vi "ConvertDataSetToWfm.vi"(10 "DataSet":T1) -> (2 "waveform":waveform(sgl))   [LabVIEW 2016]
doc: "Converts a NI InsightCM data set to a waveform data type."
uses:
  <vilib>/addons/InsightCM/Utilities/PropertyHelpers/PropertyHelpers.lvlib
  <vilib>/addons/InsightCM/MessageBus/Base/controls/KeyValuePair.ctl
  <vilib>/addons/InsightCM/MessageBus/Base/controls/DataSetByteData.ctl
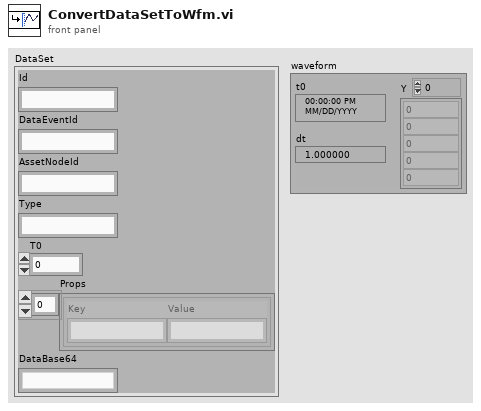
[diagram p1: front panel]
types:
  T1 = typedef "DataSetByteData.ctl" = cluster{"Id":string, "DataEventId":string, "AssetNodeId":string, "Type":string, "T0":i64, "Props":T2[], "DataBase64":string}
  T2 = typedef "KeyValuePair.ctl" = cluster{"Key":string, "Value":string}
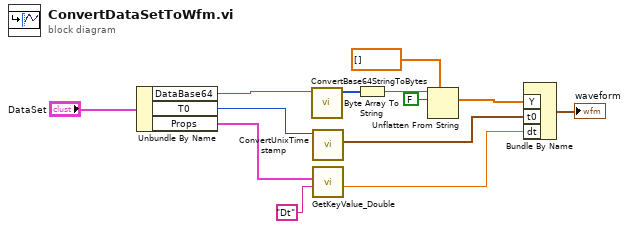
[diagram p0: block diagram]
diagram:
  n1 = Unbundle By Name("DataSet") -> ("DataBase64"=w4:string, "T0"=w2:i64, "Props"=w1:T2[])
  n2 = call <vilib>:"ConvertBase64StringToBytes.vi"("Base64 string"=w4) -> ("U8 array"=w8:u8[])  [unwired: 9 in, 1 out]
  n3 = call <vilib>:"ConvertUnixTimestamp.vi"("Timestamp in"=w2) -> ("Time Stamp out"=w12:timestamp)  [unwired: 10 in]
  n4 = call <vilib>:"GetKeyValue_Double.vi"("key"="Dt", "key value pairs"=w1) -> ("value"=w10:dbl)  [unwired: 7 in, 2 out]
  n5 = Byte Array To String(unsigned byte array=w8) -> (string=w7:string)
  n6 = Unflatten From String(type=sgl[] [], binary string=w7, data includes array or string size? (T)=FALSE) -> (value=w3:sgl[])  [unwired: 2 in, 2 out]
  n7 = Bundle By Name("Y"=w3, "t0"=w12, "dt"=w10) -> (→"waveform":waveform(sgl))  [unwired: 1 in]
